vi "Word Statistics by Any.vi"(11 "Dictionary":string[](array[string])) -> (3 "Word Statistic":T1[](array[typedef]))   [LabVIEW 2015]
uses:
  TypeDef/Word Statistic.ctl
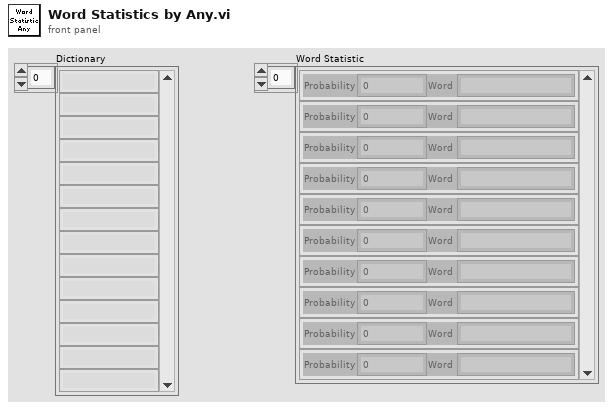
[diagram p1: front panel]
types:
  T1 = typedef "Word Statistic.ctl" = cluster{"Probability":dbl, "Word":string}
  T2 = typedef "Letter Statistic.ctl" = cluster{"Letter":string, "any":dbl, "1":dbl, "2":dbl, "3":dbl, "4":dbl, "5":dbl}
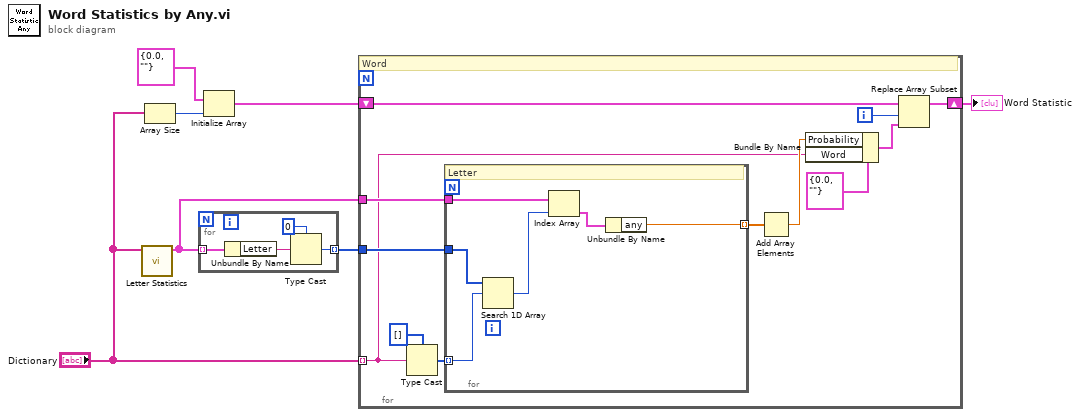
[diagram p0: block diagram]
diagram:
  n1 = call "Letter Statistics.vi"("Dictionary"="Dictionary") -> ("Statistic"=w6:T2[])  [unwired: 10 in]
  n2 = Array Size(array="Dictionary") -> (size(s)=w4:i32)
  n3 = for {
    tunnel: w6 -> [w11] mode=indexing
    tunnel: [w9] -> w7 mode=indexing
    n4 = Unbundle By Name(w11) -> ("Letter"=w8:string)
    n5 = Type Cast(type=u8 0, x=w8) -> (*(type *) &x=w9:u8)
  }
  n6 = Initialize Array(T1 {"Probability"=0.0, "Word"=""} ("Word Statistic"), w4) -> (w2:T1[])
  n7 = for {
    tunnel: "Dictionary" -> [w12] mode=indexing
    tunnel: w6 -> [w23]
    tunnel: w7 -> [w22]
    shift-right: [w17] -> w1
    shift-left: w2 -> [w18]
    i -> [w15]
    # "Word"
    n8 = Type Cast(type=u8[] [] ("letter"), x=w12) -> (*(type *) &x=w21:u8[])
    n9 = for {
      tunnel: w21 -> [w29] mode=indexing
      tunnel: w23 -> [w27]
      tunnel: w22 -> [w26]
      tunnel: [w24] -> w14 mode=indexing
      # "Letter"
      n10 = Search 1D Array(1D array=w26, element=w29) -> (index of element=w28:i32)  [unwired: 1 in]
      n11 = Index Array(array=w27, index=w28) -> (element=w25:T2)
      n12 = Unbundle By Name(w25) -> ("any"=w24:dbl)
    }
    n13 = Add Array Elements(numeric array=w14) -> (sum=w13:dbl)
    n14 = Bundle By Name(cluster=T1 {"Probability"=0.0, "Word"=""} ("Word Statistic"), "Probability"=w13, "Word"=w12) -> (w16:T1)
    n15 = Replace Array Subset(array=w18, new element=w16, index=w15) -> (w17:T1[])
  }
  "Word Statistic" <- w1
